vi "FPGA_controller.vi"() -> ()   [LabVIEW 2017]
uses:
  <vilib>/rvi/Emulation/niFpgaGetClockAttributes.vi
  <vilib>/rvi/Emulation/niFpgaSctlEmulationGetInTimedLoop.vi
  <vilib>/rvi/Emulation/niFpgaEmulationReportErrorSimple.vi
  <vilib>/rvi/eio/common/nirviEmuTemplateMethod_errors.vi
  <vilib>/rvi/Emulation/niFpgaCriticalErrorInLSC.vi
  <vilib>/eio/EIONode/EIONode.xnode
panel:
  out "Translated":i16
  out "VALID":bool
  in  "m_first u2":fxp<+/-,64,32>=-0.8999999999068677 format="%#_42g"
  in  "m_first u1":fxp<+/-,64,32>=-0.8999999999068677 format="%#_42g"
  in  "Scale u2":fxp<+/-,64,42>=5.0 format="%#_35g"
  in  "Offset u2":fxp<+/-,64,41>=2.0 format="%#_36g"
  in  "Scale u1":fxp<+/-,64,42>=5.0 format="%#_35g"
  in  "Offset u1":fxp<+/-,64,41>=2.0 format="%#_36g"
  in  "eta u":fxp<+/-,64,32>=0.30000000004656613 format="%#_42g"
  in  "Scale x2":fxp<+/-,32,16>=10.0 format="%#_21g"
  in  "m_first x2":fxp<+/-,49,33> format="%#_26g"
  in  "Offset x2":fxp<+/-,48,32> format="%#_26g"
  in  "Offset x3":fxp<+/-,48,32>=5.0 format="%#_26g"
  in  "m_first x3":fxp<+/-,32,16>=-3.399993896484375 format="%#_21g"
  in  "Scale x3":fxp<+/-,32,16>=10.0 format="%#_21g"
  in  "1/eta x":fxp<+/-,32,16>=5.0 format="%#_21g"
  in  "m_first x1":fxp<+/-,49,33> format="%#_26g"
  in  "Offset x1":fxp<+/-,48,32> format="%#_26g"
  in  "Scale x1":fxp<+/-,32,16>=10.0 format="%#_21g"
  in  "stop":bool
  # "INPUTS CONVERSION"
  # "STATES CONVERSION"
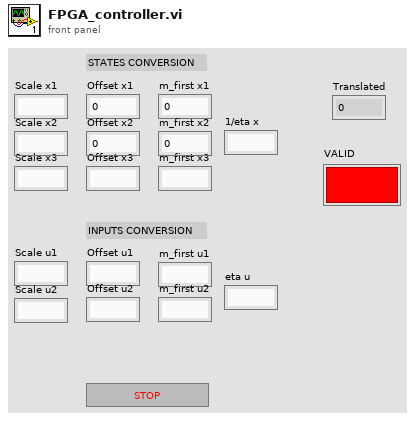
[diagram p1: front panel]
types:
  T1 = cluster{"Boolean array[0]":bool, "Boolean array[1]":bool, "Boolean array[2]":bool, "Boolean array[3]":bool, "Boolean array[4]":bool, "Boolean array[5]":bool, "Boolean array[6]":bool, "Boolean array[7]":bool, "Boolean array[8]":bool, "Boolean array[9]":bool, "Boolean array[10]":bool, "Boolean array[11]":bool, "Boolean array[12]":bool, "Boolean array[13]":bool, "Boolean array[14]":bool, "Boolean array[15]":bool, "Boolean array[16]":bool, "Boolean array[17]":bool}
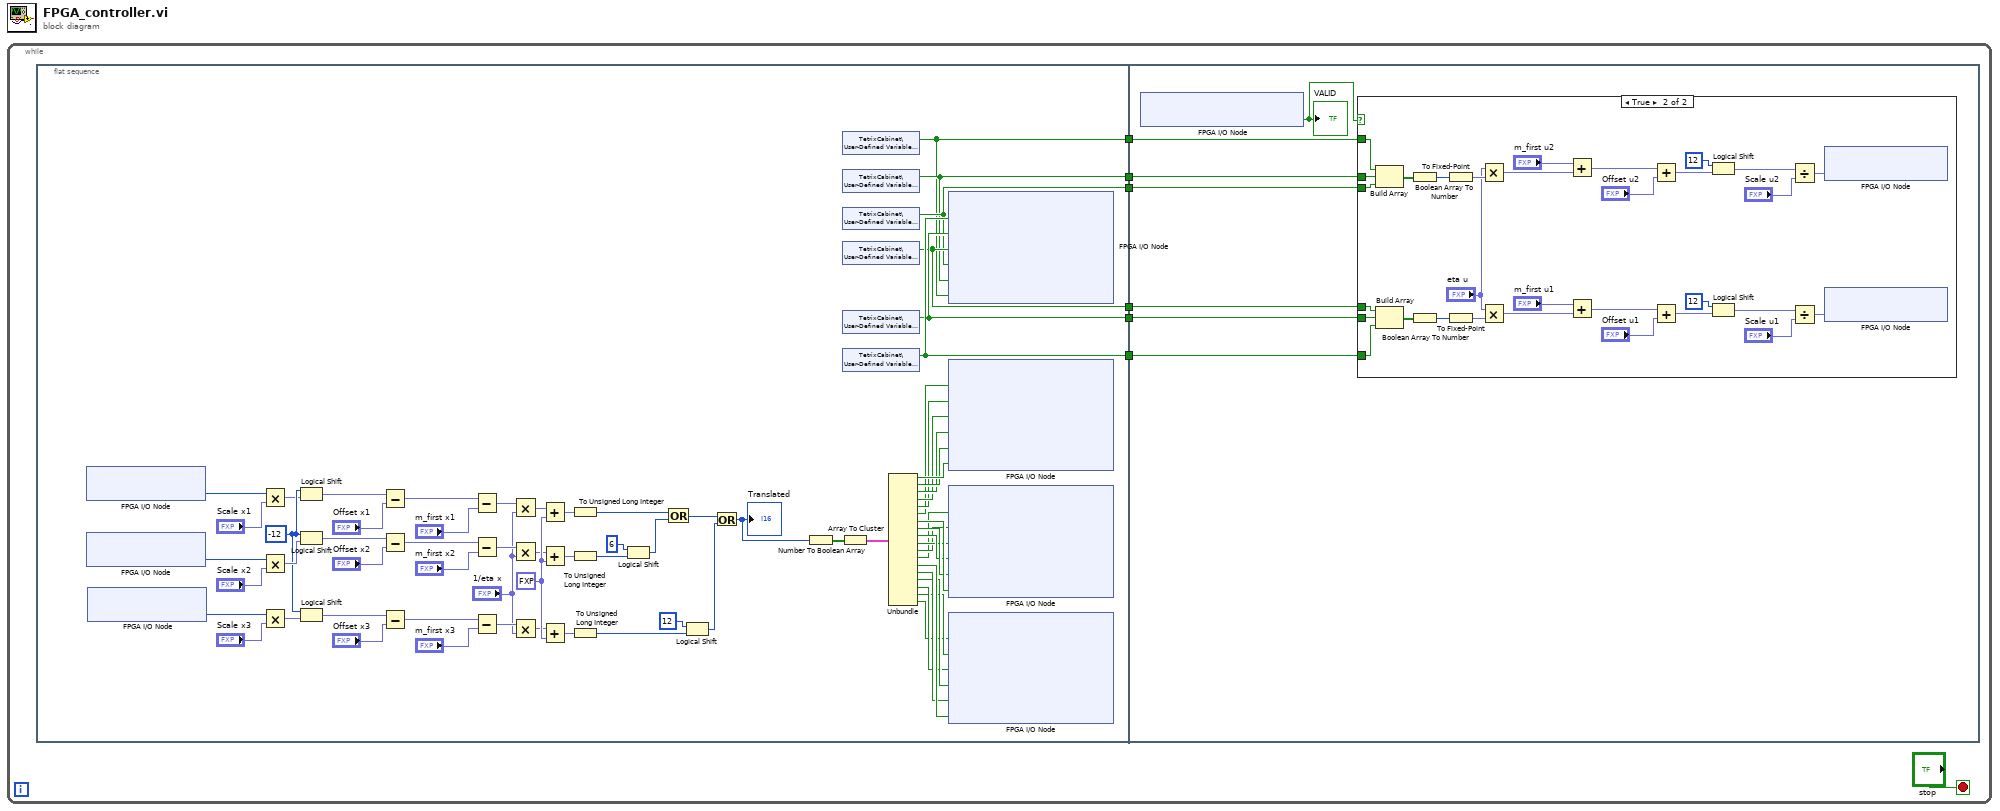
[diagram p0: block diagram]
diagram:
  n1 = while {
    stop <- "stop" stop-if-true
    n2 = flat-sequence {
      tunnel: [w13] -> w6
      tunnel: [w12] -> w5
      tunnel: [w11] -> w4
      tunnel: [w10] -> w3
      tunnel: [w9] -> w2
      tunnel: [w8] -> w1
      tunnel: w6 -> [w82]
      tunnel: w5 -> [w81]
      tunnel: w4 -> [w80]
      tunnel: w3 -> [w79]
      tunnel: w2 -> [w78]
      tunnel: w1 -> [w77]
      frame #0 {
        w45 = fxp<+/-,64,32> 0.5 ("y")
        w40 = i16 -12 ("y")
        n3 = xnode "FPGA I/O Node"() -> ("ConnectorA/AI0"=w34:u16)  [unwired: 1 in, 1 out]
        n4 = xnode "FPGA I/O Node"() -> ("ConnectorA/AI1"=w39:u16)  [unwired: 1 in, 1 out]
        n5 = xnode "FPGA I/O Node"() -> ("ConnectorB/AI0"=w38:u16)  [unwired: 1 in, 1 out]
        n6 = Multiply(x=w34, y="Scale x1") -> (x*y=w33:fxp<+/-,48,32>)
        n7 = Multiply(x=w39, y="Scale x2") -> (x*y=w46:fxp<+/-,48,32>)
        n8 = Multiply(x=w38, y="Scale x3") -> (x*y=w36:fxp<+/-,48,32>)
        n9 = Logical Shift(y=w40, x=w33) -> (x << y=w30:fxp<+/-,48,32>)
        n10 = Logical Shift(y=w40, x=w46) -> (x << y=w27:fxp<+/-,48,32>)
        n11 = Logical Shift(y=w40, x=w36) -> (x << y=w35:fxp<+/-,48,32>)
        n12 = Subtract(x=w30, y="Offset x1") -> (x-y=w31:fxp<+/-,49,33>)
        n13 = Subtract(x=w27, y="Offset x2") -> (x-y=w28:fxp<+/-,49,33>)
        n14 = Subtract(x=w35, y="Offset x3") -> (x-y=w37:fxp<+/-,49,33>)
        n15 = Subtract(x=w31, y="m_first x1") -> (x-y=w32:fxp<+/-,50,34>)
        n16 = Subtract(x=w28, y="m_first x2") -> (x-y=w26:fxp<+/-,50,34>)
        n17 = Subtract(x=w37, y="m_first x3") -> (x-y=w42:fxp<+/-,50,34>)
        n18 = Multiply(x=w32, y="1/eta x") -> (x*y=w29:fxp<+/-,64,49>)
        n19 = Multiply(x=w26, y="1/eta x") -> (x*y=w25:fxp<+/-,64,49>)
        n20 = Multiply(x=w42, y="1/eta x") -> (x*y=w41:fxp<+/-,64,49>)
        n21 = Add(x=w29, y=w45) -> (x+y=w55:fxp<+/-,64,50>)
        n22 = Add(x=w25, y=w45) -> (x+y=w44:fxp<+/-,64,50>)
        n23 = Add(x=w41, y=w45) -> (x+y=w43:fxp<+/-,64,50>)
        n24 = To Unsigned Long Integer(number=w55) -> (unsigned 32bit integer=w51:u32)
        n25 = To Unsigned Long Integer(number=w44) -> (unsigned 32bit integer=w53:u32)
        n26 = To Unsigned Long Integer(number=w43) -> (unsigned 32bit integer=w49:u32)
        n27 = Logical Shift(y=6, x=w53) -> (x << y=w52:u32)
        n28 = Or(x=w51, y=w52) -> (x .or. y?=w47:u32)
        n29 = Logical Shift(y=12, x=w49) -> (x << y=w48:u32)
        n30 = Or(x=w47, y=w48) -> (x .or. y?=w14:u32)
        "Translated" <- w14
        n31 = Number To Boolean Array(number=w14) -> (Boolean array=w56:bool[])
        n32 = Array To Cluster(array=w56) -> (cluster=w75:T1)
        n33 = shared-variable "TetrixCabinet\\User-Defined Variables\\Input_6"() -> (w8:bool)  [unwired: 1 in, 1 out]
        n34 = shared-variable "TetrixCabinet\\User-Defined Variables\\Input_5"() -> (w9:bool)  [unwired: 1 in, 1 out]
        n35 = shared-variable "TetrixCabinet\\User-Defined Variables\\Input_4"() -> (w10:bool)  [unwired: 1 in, 1 out]
        n36 = shared-variable "TetrixCabinet\\User-Defined Variables\\Input_3"() -> (w11:bool)  [unwired: 1 in, 1 out]
        n37 = shared-variable "TetrixCabinet\\User-Defined Variables\\Input_2"() -> (w12:bool)  [unwired: 1 in, 1 out]
        n38 = shared-variable "TetrixCabinet\\User-Defined Variables\\Input_1"() -> (w13:bool)  [unwired: 1 in, 1 out]
        n39 = Unbundle(w75) -> ("Boolean array[0]"=w74:bool, "Boolean array[1]"=w73:bool, "Boolean array[2]"=w72:bool, "Boolean array[3]"=w71:bool, "Boolean array[4]"=w70:bool, "Boolean array[5]"=w69:bool, "Boolean array[6]"=w68:bool, "Boolean array[7]"=w67:bool, "Boolean array[8]"=w66:bool, "Boolean array[9]"=w65:bool, "Boolean array[10]"=w64:bool, "Boolean array[11]"=w63:bool, "Boolean array[12]"=w62:bool, "Boolean array[13]"=w61:bool, "Boolean array[14]"=w60:bool, "Boolean array[15]"=w59:bool, "Boolean array[16]"=w58:bool, "Boolean array[17]"=w57:bool)
        n40 = xnode "FPGA I/O Node"("Component-Level IP\\pi18"=w13, "Component-Level IP\\pi19"=w12, "Component-Level IP\\pi20"=w11, "Component-Level IP\\pi21"=w10, "Component-Level IP\\pi22"=w9, "Component-Level IP\\pi23"=w8) -> ()  [unwired: 6 in, 6 out]
        n41 = xnode "FPGA I/O Node"("Component-Level IP\\pi00"=w69, "Component-Level IP\\pi01"=w70, "Component-Level IP\\pi02"=w71, "Component-Level IP\\pi03"=w72, "Component-Level IP\\pi04"=w73, "Component-Level IP\\pi05"=w74) -> ()  [unwired: 6 in, 6 out]
        n42 = xnode "FPGA I/O Node"("Component-Level IP\\pi06"=w63, "Component-Level IP\\pi07"=w64, "Component-Level IP\\pi08"=w65, "Component-Level IP\\pi09"=w66, "Component-Level IP\\pi10"=w67, "Component-Level IP\\pi11"=w68) -> ()  [unwired: 6 in, 6 out]
        n43 = xnode "FPGA I/O Node"("Component-Level IP\\pi12"=w57, "Component-Level IP\\pi13"=w58, "Component-Level IP\\pi14"=w59, "Component-Level IP\\pi15"=w60, "Component-Level IP\\pi16"=w61, "Component-Level IP\\pi17"=w62) -> ()  [unwired: 6 in, 6 out]
      }
      frame #1 {
        n44 = xnode "FPGA I/O Node"() -> ("Component-Level IP\\po0"=w76:bool)  [unwired: 1 in, 1 out]
        "VALID" <- w76
        n45 = case shown="True" w76 {
          tunnel: w82 -> [_ w95]
          tunnel: w81 -> [_ w94]
          tunnel: w80 -> [_ w93]
          tunnel: w79 -> [_ w92]
          tunnel: w78 -> [_ w91]
          tunnel: w77 -> [_ w90]
          frame False {
          }
          frame True {
            n46 = Build Array(w90, w91, w92) -> (w103:bool[])
            n47 = Build Array(w93, w94, w95) -> (w112:bool[])
            n48 = Boolean Array To Number(Boolean array=w103) -> (number=w101:u8)
            n49 = Boolean Array To Number(Boolean array=w112) -> (number=w110:u8)
            n50 = To Fixed-Point(number=w101) -> (fixed-point=w100:fxp<+,8,8>)  [unwired: 1 in]
            n51 = To Fixed-Point(number=w110) -> (fixed-point=w109:fxp<+,8,8>)  [unwired: 1 in]
            n52 = Multiply(x="eta u", y=w100) -> (x*y=w104:fxp<+/-,64,40>)
            n53 = Multiply(x="eta u", y=w109) -> (x*y=w113:fxp<+/-,64,40>)
            n54 = Add(x="m_first u2", y=w104) -> (x+y=w102:fxp<+/-,64,41>)
            n55 = Add(x="m_first u1", y=w113) -> (x+y=w111:fxp<+/-,64,41>)
            n56 = Add(x=w102, y="Offset u2") -> (x+y=w99:fxp<+/-,64,42>)
            n57 = Add(x=w111, y="Offset u1") -> (x+y=w108:fxp<+/-,64,42>)
            n58 = Logical Shift(y=i16 12, x=w99) -> (x << y=w97:fxp<+/-,64,42>)
            n59 = Logical Shift(y=i16 12, x=w108) -> (x << y=w106:fxp<+/-,64,42>)
            n60 = Divide(x=w97, y="Scale u2") -> (x/y=w96:fxp<+/-,64,65>)
            n61 = Divide(x=w106, y="Scale u1") -> (x/y=w105:fxp<+/-,64,65>)
            n62 = xnode "FPGA I/O Node"("ConnectorB/AO1"=w96) -> ()  [unwired: 1 in, 1 out]
            n63 = xnode "FPGA I/O Node"("ConnectorB/AO0"=w105) -> ()  [unwired: 1 in, 1 out]
          }
        }
      }
    }
  }
